vi "GV pockels secondary delay.vi"() -> ()   [LabVIEW 2017]
panel:
  out "PockelsFrameDelay_tick":u32
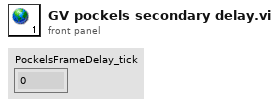
[diagram p1: front panel]
diagram:
